vi "Show Tree.vi"(7 "Root ID":string, 8 "Error In":errorcluster, 9 "Show IDs (True)":bool=TRUE, 10 "Tree Ref":refnum<vi>, 11 "Tree Manager":T1) -> (0 "Error Out":errorcluster, 3 "Tree Manager":T1)   [LabVIEW 2016, in "Tree Manager.lvclass"]
doc: "Recursively traverse down wired Tree ID and populate the Tree Control with the contents of the Tree.\n\nBecause the Tree Control requires to have only one root element, the Root ID has to be specified. This means that if you have multiple roots in your Tree you need to visualize them seperately."
uses:
  Tree Manager.lvclass
  Typedefs/Session Handle.ctl
  Tree Manager.lvclass/Tree Manager.ctl
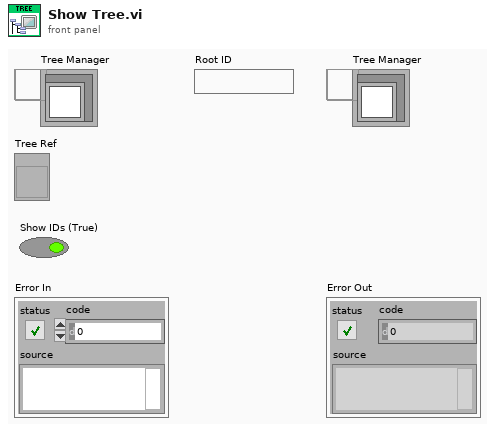
[diagram p1: front panel]
types:
  T1 = typedef "Tree Manager.lvclass/Session Handle.ctl" = refnum<data-value>
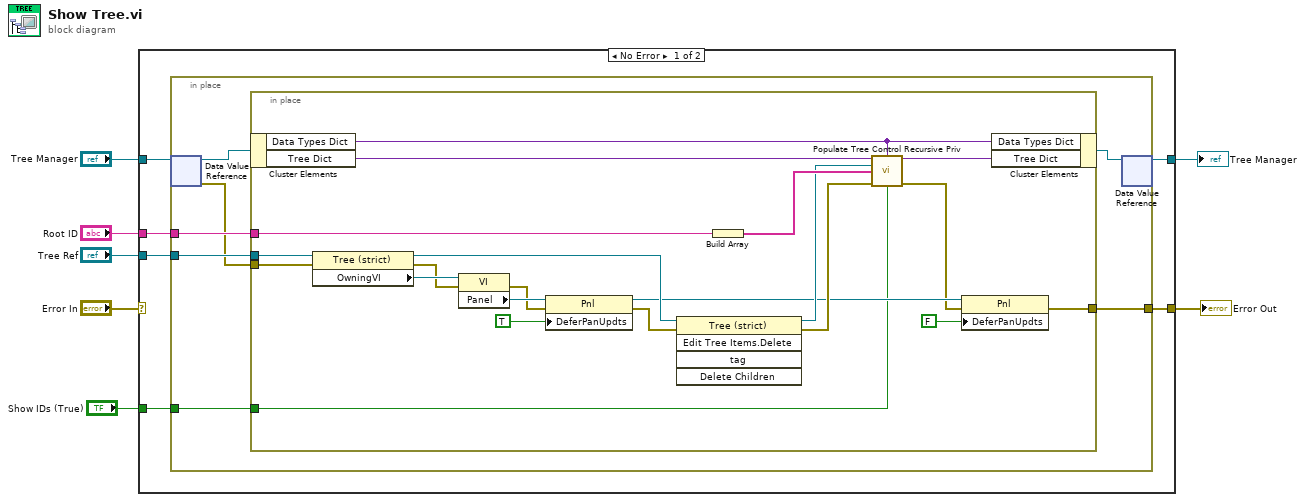
[diagram p0: block diagram]
diagram:
  n1 = case shown="No Error" "Error In" {
    selector: "Error In" -> [_ w42]
    tunnel: "Tree Manager" -> [w13 w43]
    tunnel: [w12 w43] -> w6
    tunnel: [w9 w42] -> w4
    tunnel: "Root ID" -> [w11 _]
    tunnel: "Tree Ref" -> [w10 _]
    tunnel: "Show IDs (True)" -> [w8 _]
    frame No Error {
      n2 = in-place {
        in-place-border: w11 -> [w18]
        in-place-border: w10 -> [w16]
        in-place-border: [w17] -> w9
        in-place-border: w8 -> [w14]
        n3 = in-place-dvr #1(w13) -> (w20:refnum<class "Tree Manager.lvclass">, w15:errorcluster)
        n4 = in-place {
          in-place-border: w18 -> [w38]
          in-place-border: [w24] -> w17
          in-place-border: w16 -> [w35]
          in-place-border: w15 -> [w34]
          in-place-border: w14 -> [w22]
          n5 = in-place-cluster #2(w20) -> ("Data Types Dict"=w21:variant, "Tree Dict"=w41:variant)
          n6 = property class="Tree (strict)"(reference=w35, error in=w34) -> (reference out=w29:refnum<vi>, error out=w32:errorcluster, "OwningVI"=w33:refnum<vi>)
          n7 = property class="VI"(reference=w33, error in=w32) -> (error out=w30:errorcluster, "Panel"=w31:refnum<vi>)  [unwired: 1 out]
          n8 = property class="Pnl"(reference=w31, error in=w30, "DeferPanUpdts"=TRUE ("Defer Panel Updates")) -> (reference out=w26:refnum<vi>, error out=w28:errorcluster)
          n9 = invoke class="Tree (strict)" method="Edit Tree Items.Delete"(reference=w29, error in=w28) -> (reference out=w36:refnum<vi>, error out=w39:errorcluster)  [unwired: 3 in, 3 out]
          n10 = Build Array(w38) -> (w37:string[])
          n11 = call "Populate Tree Control Recursive Priv.vi"("Tree Dictionary In"=w41, "Data Types Dict"=w21, "TreeControl In"=w36, "Child IDs"=w37, "error in"=w39, "Show IDs (True)"=w22) -> ("Tree Dictionary Out"=w40:variant, "error out"=w25:errorcluster)  [unwired: 7 in, 1 out]
          n12 = property class="Pnl"(reference=w26, error in=w25, "DeferPanUpdts"=FALSE ("Defer Panel Updates")) -> (error out=w24:errorcluster)  [unwired: 1 out]
          n13 = in-place-cluster #2("Data Types Dict"=w21, "Tree Dict"=w40) -> (w19:refnum<class "Tree Manager.lvclass">)
        }
        n14 = in-place-dvr #1(w19) -> (w12:T1)  [unwired: 1 out]
      }
    }
    frame Error {
    }
  }
  "Tree Manager" <- w6
  "Error Out" <- w4
